vi "split_state_and_arguments.vi"(10 "State:Argument":string) -> (1 "Argument":string, 3 "State":string)   [LabVIEW 2015]
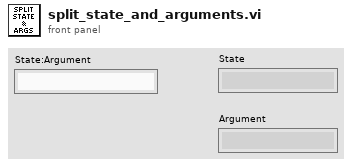
[diagram p1: front panel]
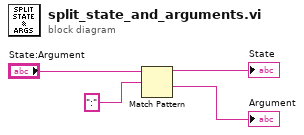
[diagram p0: block diagram]
diagram:
  n1 = Match Pattern(string="State:Argument", regular expression=":") -> (before substring=→"State":string, after substring=→"Argument":string)  [unwired: 1 in, 2 out]
